vi "Read Output.vi"(8 "error in (no error)":errorcluster, 11 "VISA resource name":refnum<visa-resource-name>) -> (0 "error out":errorcluster, 1 "Actual Current Level (0.0A)":dbl format="%.2g", 2 "Actual Voltage Level (0.0V)":dbl format="%.2g", 3 "VISA resource name out":refnum<visa-resource-name>)   [LabVIEW 2013, in "IT6900.lvlib"]
doc: "Returns the actual voltage level and actual current level for a desired channel."
uses:
  IT6900.lvlib
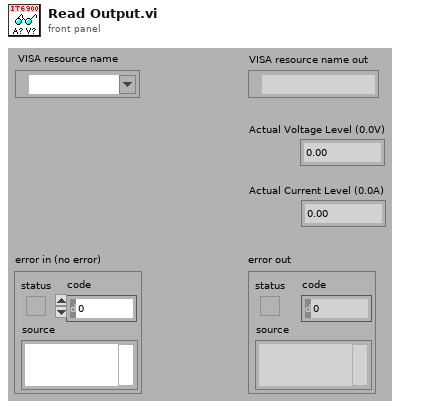
[diagram p1: front panel]
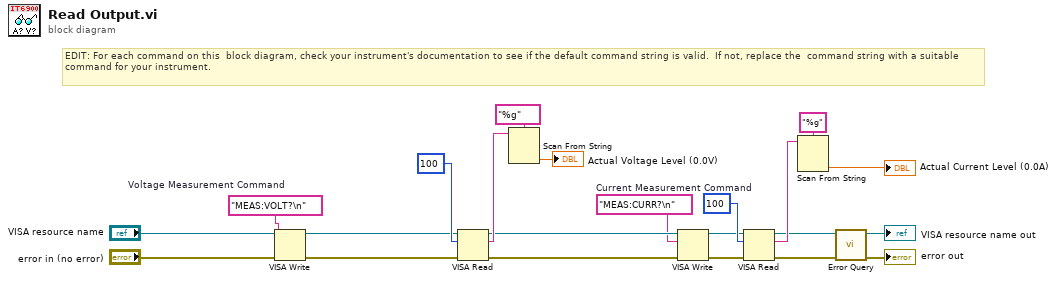
[diagram p0: block diagram]
diagram:
  w6 = "MEAS:CURR?\n"  # Current Measurement Command
  w5 = "MEAS:VOLT?\n"  # Voltage Measurement Command
  # "EDIT: For each command on this  block diagram, check your instrument's documentation to see if the default command string is valid.  If not, replace the  command string with a suitable command for your instrument."
  n1 = VISA Write(VISA resource name="VISA resource name", write buffer=w5, error in (no error)="error in (no error)") -> (VISA resource name out=w2:refnum<visa-resource-name>, error out=w1:errorcluster)  [unwired: 1 out]
  n2 = VISA Read(VISA resource name=w2, byte count=u32 100, error in (no error)=w1) -> (VISA resource name out=w7:refnum<visa-resource-name>, read buffer=w18:string, error out=w8:errorcluster)  [unwired: 1 out]
  n3 = Scan From String(format string="%g", input string=w18) -> (output 1=→"Actual Voltage Level (0.0V)":dbl)  [unwired: 3 in, 3 out]
  n4 = VISA Write(VISA resource name=w7, write buffer=w6, error in (no error)=w8) -> (VISA resource name out=w13:refnum<visa-resource-name>, error out=w12:errorcluster)  [unwired: 1 out]
  n5 = VISA Read(VISA resource name=w13, byte count=u32 100, error in (no error)=w12) -> (VISA resource name out=w10:refnum<visa-resource-name>, read buffer=w15:string, error out=w9:errorcluster)  [unwired: 1 out]
  n6 = Scan From String(format string="%g", input string=w15) -> (output 1=→"Actual Current Level (0.0A)":dbl)  [unwired: 3 in, 3 out]
  n7 = call "Error Query.vi"("error in (no error)"=w9, "VISA resource name"=w10) -> ("error out"=→"error out":errorcluster, "VISA resource name out"=→"VISA resource name out":refnum<visa-resource-name>)  [unwired: 6 in, 2 out]
